vi "JoystickControls.vi"() -> (3 "input cluster 2":T1)   [LabVIEW 2015]
uses:
  Controls.ctl
  References/Refnums.vi
  <vilib>/Rock Robotics/WPI/Utilities/WPI_GetSetVariantRefNum.vi
panel:
  out "input cluster":T1
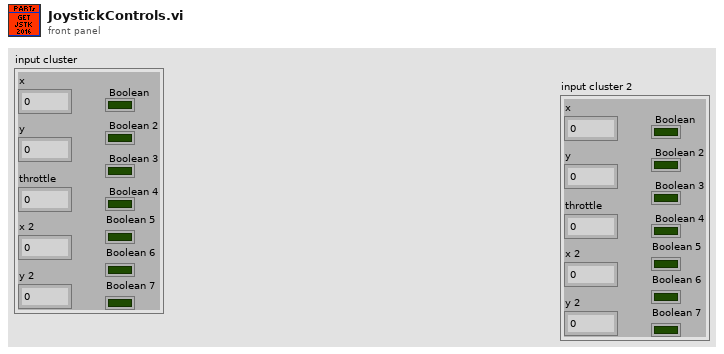
[diagram p1: front panel]
types:
  T1 = typedef "Controls.ctl" = cluster{"x":dbl, "y":dbl, "throttle":dbl, "x 2":dbl, "y 2":dbl, "Boolean":bool, "Boolean 2":bool, "Boolean 3":bool, "Boolean 4":bool, "Boolean 5":bool, "Boolean 6":bool, "Boolean 7":bool}
  T2 = typedef "WPI_JoystickDevRef.ctl" = cluster{"Device":T3}
  T3 = typedef "WPI_JoystickDeviceEnum.ctl" = enum16{"USB 0", "USB 1", "USB 2", "USB 3", "USB 4", "USB 5"}
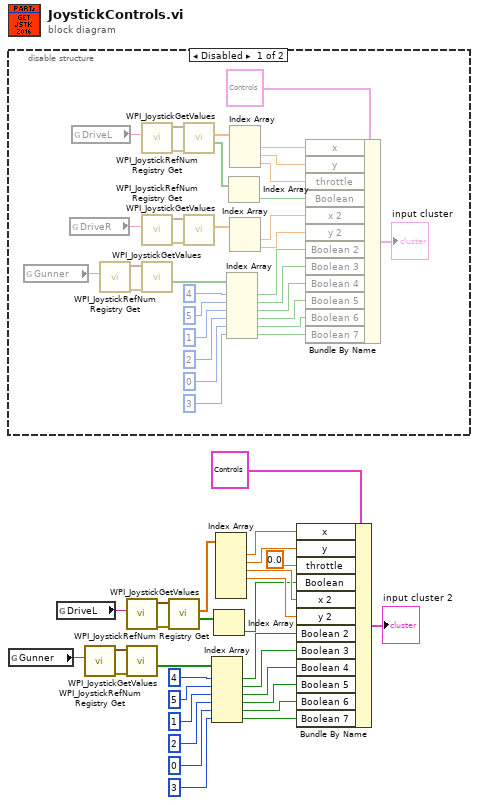
[diagram p0: block diagram]
diagram:
  n1 = disable-structure shown="Disabled" {
    frame Disabled {
      n2 = global read "Refnums.vi" "Gunner"() -> (w43:string)
      n3 = global read "Refnums.vi" "DriveR"() -> (w62:string)
      n4 = global read "Refnums.vi" "DriveL"() -> (w55:string)
      n5 = call <vilib>:"WPI_JoystickRefNum Registry Get.vi"("refnum name"=w43) -> ("error out"=w45:errorcluster, "JoystickDevRef"=w44:T2)  [unwired: 9 in]
      n6 = call <vilib>:"WPI_JoystickRefNum Registry Get.vi"("refnum name"=w55) -> ("error out"=w61:errorcluster, "JoystickDevRef"=w60:T2)  [unwired: 9 in]
      n7 = call <vilib>:"WPI_JoystickRefNum Registry Get.vi"("refnum name"=w62) -> ("error out"=w58:errorcluster, "JoystickDevRef"=w59:T2)  [unwired: 9 in]
      n8 = call <vilib>:"WPI_JoystickGetValues.vi"("error in (no error)"=w45, "JoystickDevRef"=w44) -> ("Buttons"=w42:bool[])  [unwired: 5 in, 4 out]
      n9 = call <vilib>:"WPI_JoystickGetValues.vi"("error in (no error)"=w61, "JoystickDevRef"=w60) -> ("Buttons"=w50:bool[], "Axes"=w54:dbl[])  [unwired: 5 in, 3 out]
      n10 = call <vilib>:"WPI_JoystickGetValues.vi"("error in (no error)"=w58, "JoystickDevRef"=w59) -> ("Axes"=w48:dbl[])  [unwired: 5 in, 4 out]
      n11 = Index Array(array=w42, index #1=4 ("index"), index #2=5 ("index"), index #3=1 ("index"), index #4=2 ("index"), index #5=0 ("index"), index #6=3 ("index")) -> (element #1=w41:bool, element #2=w40:bool, element #3=w39:bool, element #4=w38:bool, element #5=w37:bool, element #6=w36:bool)
      n12 = Index Array(array=w50) -> (element=w49:bool)  [unwired: 1 in]
      n13 = Index Array(array=w54) -> (element #1=w53:dbl, element #2=w52:dbl, element #3=w51:dbl)  [unwired: 3 in]
      n14 = Index Array(array=w48) -> (element #1=w47:dbl, element #2=w46:dbl)  [unwired: 2 in]
      n15 = Bundle By Name(cluster=T1 {"x"=0.0, "y"=0.0, "throttle"=0.0, "x 2"=0.0, "y 2"=0.0, "Boolean"=FALSE, "Boolean 2"=FALSE, "Boolean 3"=FALSE, "Boolean 4"=FALSE, "Boolean 5"=FALSE, "Boolean 6"=FALSE, "Boolean 7"=FALSE} ("input cluster"), "x"=w53, "y"=w52, "throttle"=w51, "Boolean"=w49, "x 2"=w47, "y 2"=w46, "Boolean 2"=w41, "Boolean 3"=w40, "Boolean 4"=w39, "Boolean 5"=w38, "Boolean 6"=w37, "Boolean 7"=w36) -> (→"input cluster":T1)
    }
    frame Enabled {
    }
  }
  n16 = global read "Refnums.vi" "Gunner"() -> (w16:string)
  n17 = global read "Refnums.vi" "DriveL"() -> (w11:string)
  n18 = call <vilib>:"WPI_JoystickRefNum Registry Get.vi"("refnum name"=w16) -> ("error out"=w14:errorcluster, "JoystickDevRef"=w15:T2)  [unwired: 9 in]
  n19 = call <vilib>:"WPI_JoystickRefNum Registry Get.vi"("refnum name"=w11) -> ("error out"=w9:errorcluster, "JoystickDevRef"=w10:T2)  [unwired: 9 in]
  n20 = call <vilib>:"WPI_JoystickGetValues.vi"("error in (no error)"=w14, "JoystickDevRef"=w15) -> ("Buttons"=w17:bool[])  [unwired: 5 in, 4 out]
  n21 = call <vilib>:"WPI_JoystickGetValues.vi"("error in (no error)"=w9, "JoystickDevRef"=w10) -> ("Buttons"=w3:bool[], "Axes"=w8:dbl[])  [unwired: 5 in, 3 out]
  n22 = Index Array(array=w17, index #1=4 ("index"), index #2=5 ("index"), index #3=1 ("index"), index #4=2 ("index"), index #5=0 ("index"), index #6=3 ("index")) -> (element #1=w18:bool, element #2=w19:bool, element #3=w20:bool, element #4=w21:bool, element #5=w22:bool, element #6=w23:bool)
  n23 = Index Array(array=w3) -> (element=w2:bool)  [unwired: 1 in]
  n24 = Index Array(array=w8) -> (element #1=w7:dbl, element #2=w6:dbl, element #3=w5:dbl, element #4=w4:dbl)  [unwired: 6 in, 2 out]
  n25 = Bundle By Name(cluster=T1 {"x"=0.0, "y"=0.0, "throttle"=0.0, "x 2"=0.0, "y 2"=0.0, "Boolean"=FALSE, "Boolean 2"=FALSE, "Boolean 3"=FALSE, "Boolean 4"=FALSE, "Boolean 5"=FALSE, "Boolean 6"=FALSE, "Boolean 7"=FALSE} ("input cluster"), "x"=w7, "y"=w6, "throttle"=0.0, "Boolean"=w2, "x 2"=w5, "y 2"=w4, "Boolean 2"=w18, "Boolean 3"=w19, "Boolean 4"=w20, "Boolean 5"=w21, "Boolean 6"=w22, "Boolean 7"=w23) -> (→"input cluster 2":T1)
